vi "read hits subvi.vi"(8 "error in (no error)":errorcluster, 10 "buffer in":T2, 11 ".NET Refnum in":T1) -> (0 "error out":errorcluster, 1 "buffer out":T2, 2 "ReadHPTDCHit":i32, 3 ".NET Refnum out":T1)   [LabVIEW 2016, in "HPTDC Driver Library.lvlib"]
uses:
  HPTDC Driver Library.lvlib
  Typedefs/TDCHitObjBuffer.ctl
  C:/Users/CRT Controller/CRTC Labview Application/Source/HPTDC Driver Library Folder/Library files/hptdc_net4_3.7.0_x64.dll
  hptdc_net4_3.7.0_x64.dll
  Typedefs/TDCManager.ctl
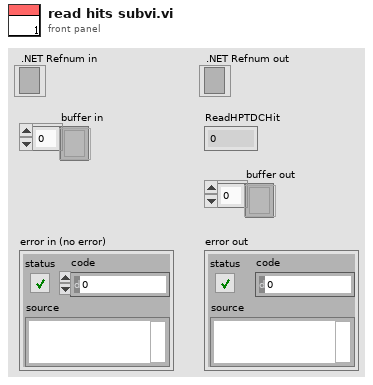
[diagram p1: front panel]
types:
  T1 = typedef "HPTDC Driver Library.lvlib/TDCManager.ctl" = refnum<k24>
  T2 = typedef "TDCHitObjBuffer.ctl" = refnum<k24>[]
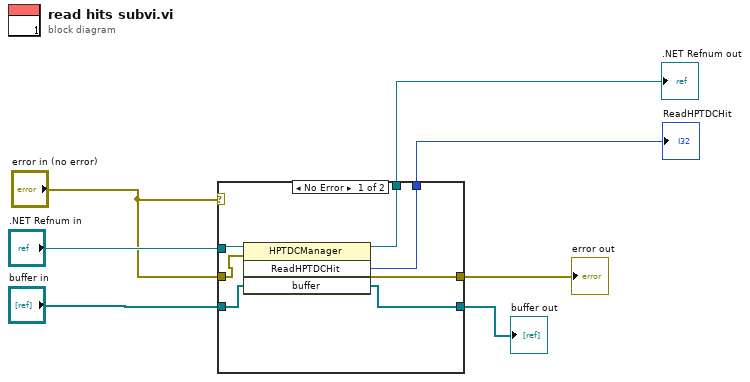
[diagram p0: block diagram]
diagram:
  n1 = case shown="No Error" "error in (no error)" {
    tunnel: "error in (no error)" -> [w10 w17]
    tunnel: "buffer in" -> [w8 w16]
    tunnel: [w9 w16] -> w6
    tunnel: [w12 w17] -> w5
    tunnel: [w11 _] -> w4
    tunnel: [w13 w15] -> w3
    tunnel: ".NET Refnum in" -> [w14 w15]
    frame No Error {
      n2 = invoke class="HPTDCManager" method="ReadHPTDCHit"(reference=w14, error in=w10, "buffer"=w8) -> (reference out=w13:T1, error out=w12:errorcluster, "ReadHPTDCHit"=w11:i32, "buffer"=w9:refnum<k24>[])  [unwired: 1 in]
    }
    frame Error {
    }
  }
  "buffer out" <- w6
  "error out" <- w5
  "ReadHPTDCHit" <- w4
  ".NET Refnum out" <- w3
